vi "DAQmx task create-Pockels modulation clock.vi"(8 "error in":errorcluster, 9 "Setup/Logging queue element":T1={"Imaging Protocol"=enum."Live Imaging", "Number of Trials"=0, "Frame Size"=512, "# Averaged frames"=0, "Dwell time (us)"=0.0, "Index of Z-plane"=0, "Timelapse?"=FALSE, "Logging process is active"=FALSE, "Speed logging enabled"=FALSE, "tdms file ref"=refnum, "path"=path "", "Trial Number"=0, "Expected # points acquired"=FALSE, "Manually stopped"=FALSE, "Last trial"=FALSE, "Ch0 data"=[], "Ch1 data"=[], "Ref Data"=[], "Ref Frame Time"=[], "Image Time"=[], "Continuous Time"=[], "Ref X Length"=0, "Ref Y Length"=0, "# Ref Averaged frames"=0, "Ref Dwell time (us)"=0.0, "Points acquired"={"Ch0 last trial"=0, "Ch1 last trial"=0, "All trials"=0}, "HW Timings File"=refnum} {"Ref Dwell time (us)" format="%#.6g"; "Frame Size" items=["100X100"=100, "128X128"=128, "200X200"=200, "256X256"=256, "512X512"=512, "1024x1024"=1024, "2048x2048"=2048]; "Dwell time (us)" format="%#.6g"}, 11 "Data length":i32) -> (0 "error out":errorcluster, 3 "Refnum out":refnum<k21>)   [LabVIEW 2020]
uses:
  Typedefs/Logging queue element.ctl
  Typedefs/Imaging Protocols enum.ctl
  Typedefs/Frame Size.ctl
  Typedefs/Acquired points count.ctl
  Global Variables/General Globals.vi
  <vilib>/DAQmx/create/channels.llb/DAQmx Create Channel (CO-Pulse Generation-Frequency).vi
  <vilib>/DAQmx/configure/timing.llb/DAQmx Timing (Implicit).vi
  <vilib>/DAQmx/configure/trigger.llb/DAQmx Start Trigger (Digital Edge).vi
  <resource>/objmgr/daqmx.rc
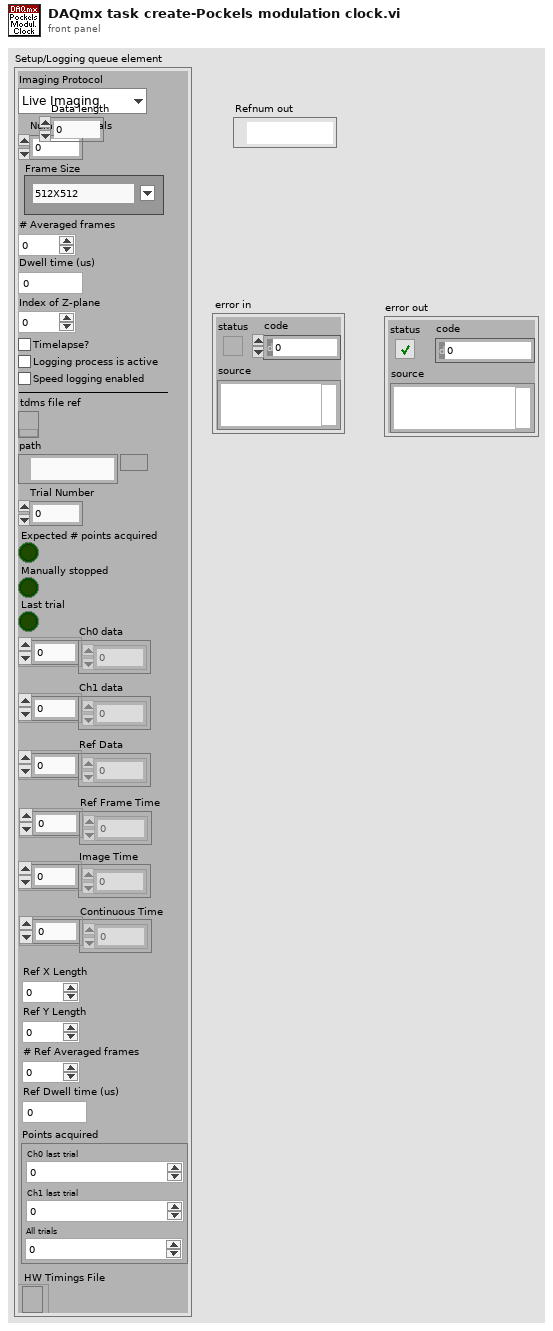
[diagram p1: front panel]
types:
  T1 = typedef "Logging queue element.ctl" = cluster{"Imaging Protocol":T2, "Number of Trials":u16, "Frame Size":T3, "# Averaged frames":u16, "Dwell time (us)":dbl, "Index of Z-plane":i32, "Timelapse?":bool, "Logging process is active":bool, "Speed logging enabled":bool, "tdms file ref":refnum<k34>, "path":path, "Trial Number":i32, "Expected # points acquired":bool, "Manually stopped":bool, "Last trial":bool, "Ch0 data":u32[], "Ch1 data":u32[], "Ref Data":u32[], "Ref Frame Time":u64[], "Image Time":u64[], "Continuous Time":u64[], "Ref X Length":u16, "Ref Y Length":u16, "# Ref Averaged frames":u16, "Ref Dwell time (us)":dbl, "Points acquired":T4, "HW Timings File":refnum<file>}
  T2 = typedef "Imaging Protocols enum.ctl" = enum16{"AOL Z-Stack", "Motor Z Stack", "Functional Acquisition", "Single Plane Acquisition", "Volume Acquisition", "Live Imaging", "Live Plane Imaging", "Live Volume Imaging"}
  T3 = typedef "Frame Size.ctl" = u16
  T4 = typedef "Acquired points count.ctl" = cluster{"Ch0 last trial":u64, "Ch1 last trial":u64, "All trials":u64}
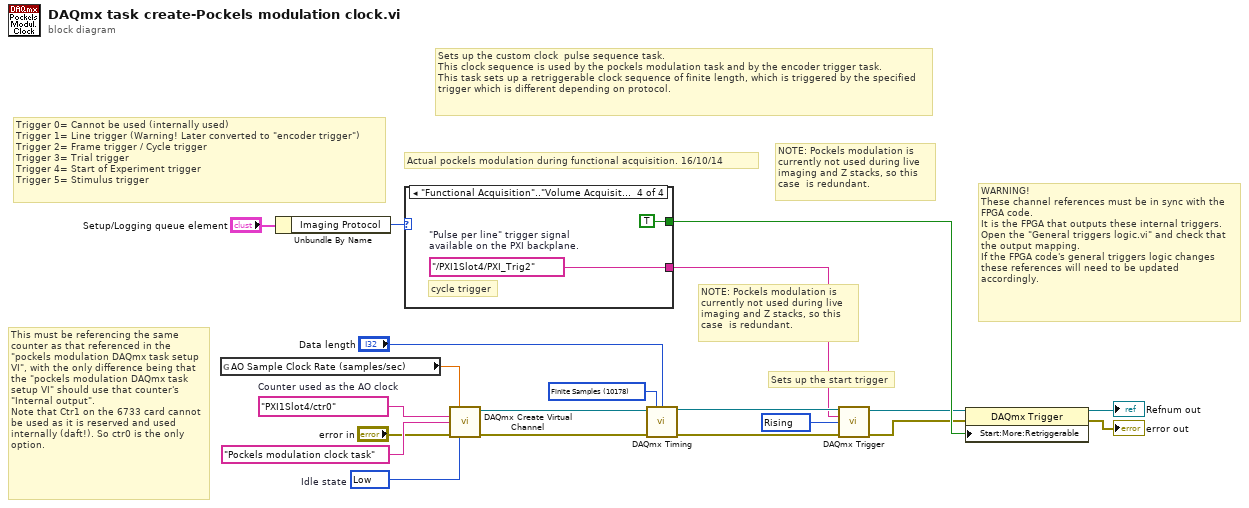
[diagram p0: block diagram]
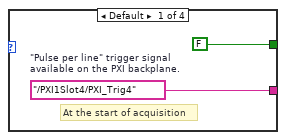
[diagram p2: hidden frame]
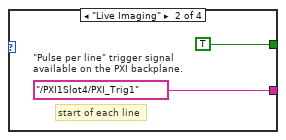
[diagram p3: hidden frame]
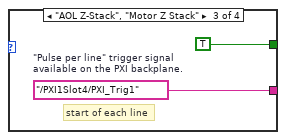
[diagram p4: hidden frame]
diagram:
  w10 = 10280 items=["Rising"=10280, "Falling"=10171] ("Trigger Edge")
  w3 = tag "PXI1Slot4/ctr0"  # Counter used as the AO clock
  w13 = 10214 items=["High"=10192, "Low"=10214]  # Idle state
  w14 = 10178 items=["Finite Samples"=10178, "Continuous Samples"=10123] ("sample mode")
  # "NOTE: Pockels modulation is currently not used during live imaging and Z stacks, so this case  is redundant."
  # "NOTE: Pockels modulation is currently not used during live imaging and Z stacks, so this case  is redundant."
  # "WARNING!\nThese channel references must be in sync with the FPGA code.\nIt is the FPGA that outputs these internal triggers. Open the \"General triggers logic.vi\" and check that the output mapping.\nIf the FPGA code's general triggers logic changes these references will need to be updated accordingly."
  # "Trigger 0= Cannot be used (internally used)\nTrigger 1= Line trigger (Warning! Later converted to \"encoder trigger\")\nTrigger 2= Frame trigger / Cycle trigger\nTrigger 3= Trial trigger\nTrigger 4= Start of Experiment trigger\nTrigger 5= Stimulus trigger"
  # "Sets up the start trigger"
  # "Sets up the custom clock  pulse sequence task.\nThis clock sequence is used by the pockels modulation task and by the encoder trigger task.\nThis task sets up a retriggerable clock sequence of finite length, which is triggered by the specified trigger which is different depending on protocol."
  # "Actual pockels modulation during functional acquisition. 16/10/14"
  # "This must be referencing the same counter as that referenced in the \"pockels modulation DAQmx task setup VI\", with the only difference being that the \"pockels modulation DAQmx task setup VI\" should use that counter's \"Internal output\".\nNote that Ctr1 on the 6733 card cannot be used as it is reserved and used internally (daft!). So ctr0 is the only option."
  n1 = global read "General Globals.vi" "AO Sample Clock Rate (samples/sec)"() -> (w1:dbl)
  n2 = Unbundle By Name("Setup/Logging queue element") -> ("Imaging Protocol"=w19:T2)
  n3 = case shown="\"Functional Acquisition\"..\"Volume Acquisition\"" w19 {
    tunnel: [FALSE TRUE TRUE TRUE] -> w20
    tunnel: [w21 w23 w25 w27] -> w2
    frame Default {
      w21 = tag "/PXI1Slot4/PXI_Trig4"  # "Pulse per line" trigger signal available on the PXI backplane.
      # "At the start of acquisition"
    }
    frame "Live Imaging" {
      w23 = tag "/PXI1Slot4/PXI_Trig1"  # "Pulse per line" trigger signal available on the PXI backplane.
      # "start of each line"
    }
    frame "AOL Z-Stack", "Motor Z Stack" {
      w25 = tag "/PXI1Slot4/PXI_Trig1"  # "Pulse per line" trigger signal available on the PXI backplane.
      # "start of each line"
    }
    frame "Functional Acquisition".."Volume Acquisition" {
      w27 = tag "/PXI1Slot4/PXI_Trig2"  # "Pulse per line" trigger signal available on the PXI backplane.
      # "cycle trigger"
    }
  }
  n4 = call-poly <vilib>:"DAQmx Create Virtual Channel.vi"("frequency"=w1, "counter"=w3, "name to assign"="Pockels modulation clock task", "error in"="error in", "idle state"=w13) -> ("task out"=w15:refnum<k21>, "error out"=w16:errorcluster)  [unwired: 9 in]
  n5 = call-poly <vilib>:"DAQmx Timing.vi"("task/channels in"=w15, "sample mode"=w14, "samples per channel"="Data length", "error in"=w16) -> ("task out"=w12:refnum<k21>, "error out"=w11:errorcluster)  [unwired: 10 in]
  n6 = call-poly <vilib>:"DAQmx Trigger.vi"("task/channels in"=w12, "source"=w2, "edge"=w10, "error in"=w11) -> ("task out"=w9:refnum<k21>, "error out"=w7:errorcluster)  [unwired: 10 in]
  n7 = property on="Property Node" class="DAQmx Trigger"(reference=w9, error in=w7, "Start:More:Retriggerable"=w20) -> (reference out=→"Refnum out":refnum<k21>, error out=→"error out":errorcluster)
